vi "SERVO_DEG_OUT_2.vi"(0 "VISA Refnum in":refnum<visa-resource-name>, 1 "Voltage":u16, 2 "Flush after read":bool=TRUE, 3 "error in (no error)":errorcluster) -> (7 "VISA Refnum out":refnum<visa-resource-name>, 8 "Actual Set Voltage":dbl format="%_9g", 10 "error out":errorcluster)   [LabVIEW 2023]
uses:
  <vilib>/Utility/error.llb/Error Cluster From Error Code.vi
  <vilib>/regexp/Match Regular Expression.xnode
  <vilib>/ErrorRing/Error Ring.xnode
panel:
  out "String":string
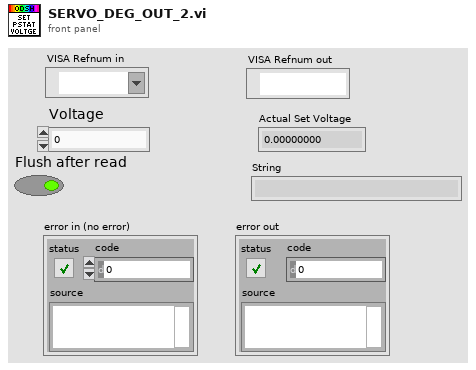
[diagram p1: front panel]
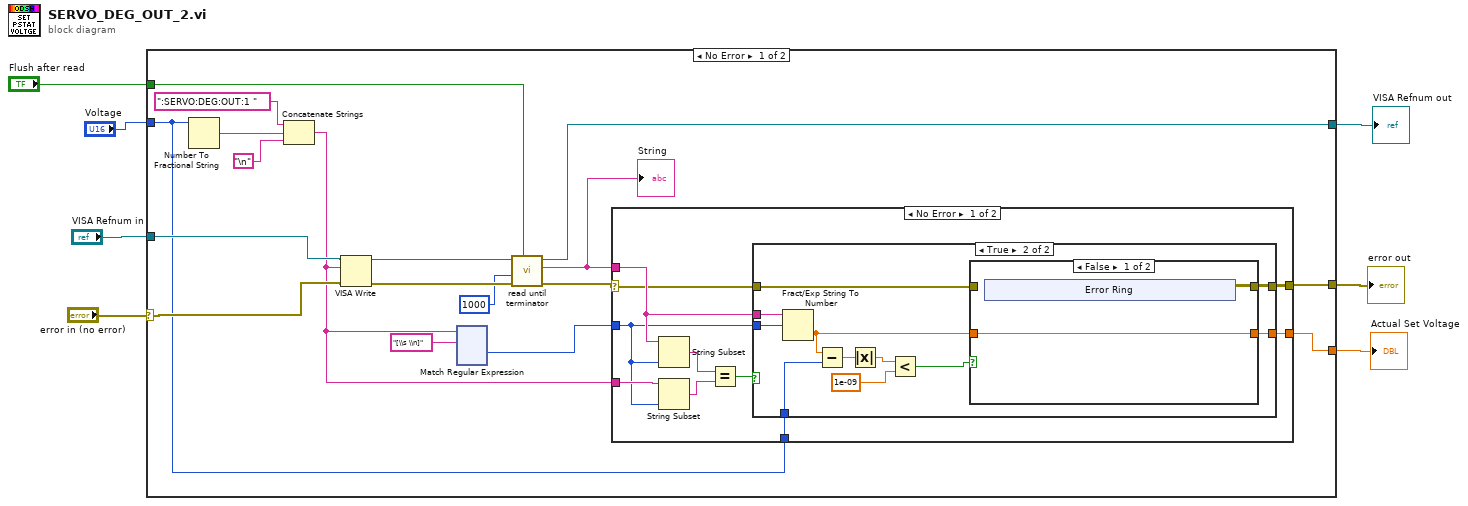
[diagram p0: block diagram]
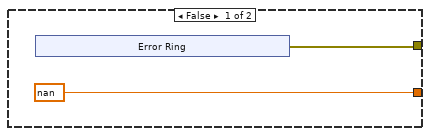
[diagram p2: hidden frame]
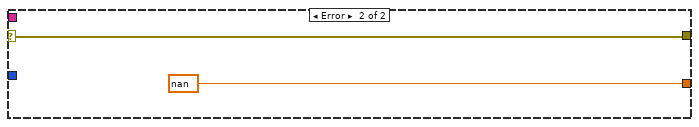
[diagram p4: hidden frame]
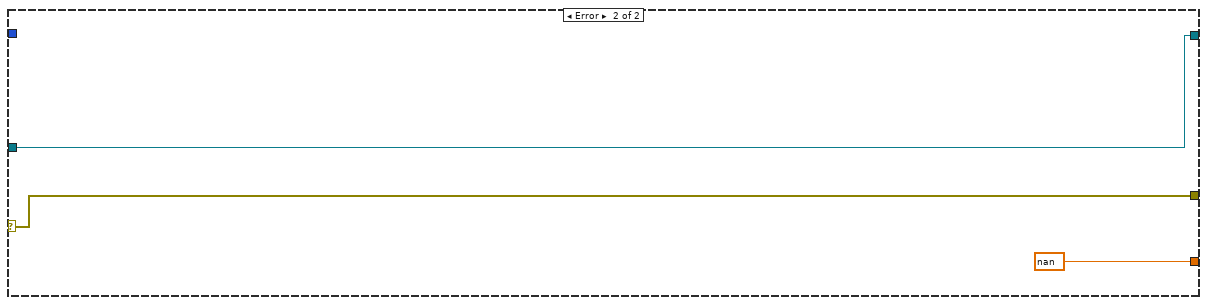
[diagram p5: hidden frame]
diagram:
  n1 = case shown="No Error" "error in (no error)" {
    selector: "error in (no error)" -> [w14 w184]
    tunnel: "VISA Refnum in" -> [w25 w183]
    tunnel: [w22 w183] -> w6
    tunnel: [w20 nan] -> w5
    tunnel: [w18 w184] -> w4
    tunnel: "Voltage" -> [w9 _]
    tunnel: "Flush after read" -> [w8 _]
    frame No Error {
      n2 = Number To Fractional String(number=w9) -> (F-format string=w10:string)  [unwired: 3 in]
      n3 = Concatenate Strings(":SERVO:DEG:OUT:1 " ("buffer d'écriture"), w10, "\n") -> (w11:string)
      n4 = VISA Write(VISA resource name=w25, write buffer=w11, error in (no error)=w14) -> (VISA resource name out=w24:refnum<visa-resource-name>, error out=w23:errorcluster)  [unwired: 1 out]
      n5 = xnode "Match Regular Expression"("chaîne en entrée"=w11, "expression régulière"="[\\s \\n]" ("regular expression")) -> ("offset après correspondance"=w15:i32)  [unwired: 4 in, 4 out]
      n6 = call "read until terminator.vi"("Flush after read"=w8, "error in (no error)"=w23, "Timeout (ms)"=1000, "VISA Refnum in"=w24) -> ("error out"=w19:errorcluster, "String"=w17:string, "VISA Refnum out"=w22:refnum<visa-resource-name>)  [unwired: 5 in]
      "String" <- w17
      n7 = case shown="No Error" w19 {
        selector: w19 -> [w145 w180]
        tunnel: w17 -> [w150 _]
        tunnel: [w152 nan] -> w20
        tunnel: [w144 w180] -> w18
        tunnel: w15 -> [w149 _]
        tunnel: w11 -> [w151 _]
        tunnel: w9 -> [w143 _]
        frame No Error {
          n8 = String Subset(string=w150, length (rest)=w149) -> (substring=w148:string)  [unwired: 1 in]
          n9 = String Subset(string=w151, length (rest)=w149) -> (substring=w147:string)  [unwired: 1 in]
          n10 = Equal?(x=w148, y=w147) -> (x = y?=w146:bool)
          n11 = case shown="True" w146 {
            tunnel: [nan w166] -> w152
            tunnel: w150 -> [_ w170]
            tunnel: w149 -> [_ w169]
            tunnel: w145 -> [_ w168]
            tunnel: [w153 w167] -> w144
            tunnel: w143 -> [_ w164]
            frame False {
              n12 = xnode "Error Ring"() -> ("error out"=w153:errorcluster)
            }
            frame True {
              n13 = Fract/Exp String To Number(string=w170, offset=w169) -> (number=w165:dbl)  [unwired: 2 in, 1 out]
              n14 = Subtract(x=w165, y=w164) -> (x-y=w163:dbl)
              n15 = Absolute Value(x=w163) -> (abs(x)=w162:dbl)
              n16 = Less?(x=w162, y=1e-09) -> (x < y?=w160:bool)
              n17 = case shown="False" w160 {
                tunnel: w168 -> [_ w179]
                tunnel: [w171 w179] -> w167
                tunnel: w165 -> [w172 w178]
                tunnel: [w172 w178] -> w166
                frame False {
                  n18 = xnode "Error Ring"() -> ("error out"=w171:errorcluster)
                }
                frame True {
                }
              }
            }
          }
        }
        frame Error {
        }
      }
    }
    frame Error {
    }
  }
  "error out" <- w4
  "VISA Refnum out" <- w6
  "Actual Set Voltage" <- w5
